vi "Create.vi"(8 "error in (no error)":errorcluster, 9 "Gun VRML":string="content/models/mp5r.wrl", 10 "Position":T1={"X"=-4.0, "Y"=2.0, "Z"=4.0}) -> (0 "error out":errorcluster, 2 "Model":refnum<class "3D Object.lvclass">, 3 "Player out":refnum<class "Player.lvclass">)   [LabVIEW 2015, in "Player.lvclass"]
uses:
  Player.lvclass
  3D Point.ctl
  3D Object/3D Object.lvclass
  Player.lvclass/Player.ctl
  3D Object/Object.vi
  3D Object/VRML.vi
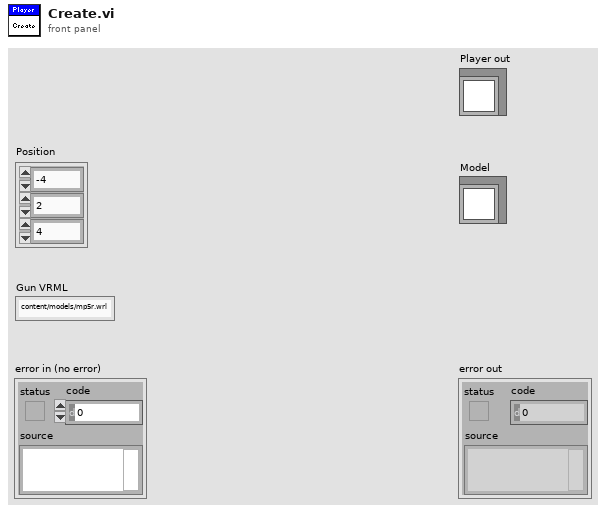
[diagram p1: front panel]
types:
  T1 = typedef "3D Point.ctl" = cluster{"X":sgl, "Y":sgl, "Z":sgl}
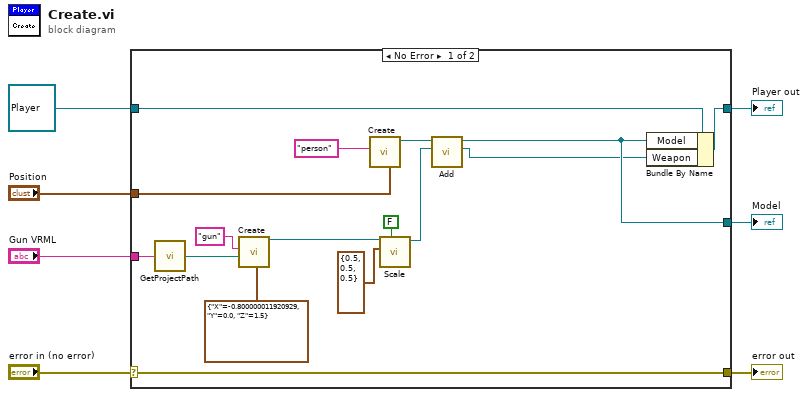
[diagram p0: block diagram]
diagram:
  n1 = case shown="No Error" "error in (no error)" {
    selector: "error in (no error)" -> [w23 w25]
    tunnel: [w23 w25] -> w6
    tunnel: [w11 w24] -> w4
    tunnel: refnum<class "Player.lvclass"> refnum ("Player in") -> [w12 w24]
    tunnel: "Gun VRML" -> [w14 _]
    tunnel: "Position" -> [w13 _]
    tunnel: [w10 _] -> w1
    frame No Error {
      n2 = call "GetProjectPath.vi"("File"=w14) -> ("Path"=w17:path)
      n3 = call-poly "Create.vi"("Position"=cluster{"X":sgl, "Y":sgl, "Z":sgl} {"X"=-0.8, "Y"=0.0, "Z"=1.5}, "Path"=w17, "Name"="gun") -> ("3D Object out"=w22:refnum<class "3D Object.lvclass">)  [unwired: 7 in, 1 out]
      n4 = call-poly "Create.vi"("Position"=w13, "Name"="person") -> ("3D Object out"=w18:refnum<class "3D Object.lvclass">)  [unwired: 8 in, 1 out]
      n5 = call "Scale.vi"("Relative?"=FALSE, "Scale"=cluster{"Z":sgl, "Y":sgl, "X":sgl} {"Z"=0.5, "Y"=0.5, "X"=0.5}, "3D Object in"=w22) -> ("3D Object out"=w8:refnum<class "3D Object.lvclass">)  [unwired: 7 in, 1 out]
      n6 = call "Add.vi"("Child in"=w8, "Parent in"=w18) -> ("Child out"=w9:refnum<class "3D Object.lvclass">, "Parent out"=w10:refnum<class "3D Object.lvclass">)  [unwired: 7 in, 1 out]
      n7 = Bundle By Name(cluster=w12, "Model"=w10, "Weapon"=w9) -> (w11:refnum<class "Player.lvclass">)
    }
    frame Error {
    }
  }
  "error out" <- w6
  "Player out" <- w4
  "Model" <- w1
